vi "DataSelectNew.vi"(8 "error in (no error)":errorcluster, 9 "Table":string, 11 "Machine":string) -> (2 "error out":errorcluster)   [LabVIEW 2012]
uses:
  <vilib>/addons/database/Auxilliary.llb/DB Tools Cursor Type.ctl
  Global1.vi
  <vilib>/addons/database/Connection.llb/DB Tools Open Connec (Path).vi
  <vilib>/addons/database/Connection.llb/Conn Execute.vi
  <vilib>/addons/database/Recordset.llb/Rec Fetch Integer Data (R).vi
  <vilib>/addons/database/Recordset.llb/Rec Destroy - Connection.vi
  <vilib>/addons/database/_DB Variant To Data/Database Variant To Data.xnode
  <vilib>/addons/database/NI_Database_API.lvlib
panel:
  out "concatenated string 3":string
  out "error out 3":errorcluster
  out "data 3":i32
  out "concatenated string 2":string
  out "x > y?":bool
  out "concatenated string":string
  in  "input cluster":T1
  out "sum 2":i32
  in  "input cluster 2":T1
  out "sum":i32
  out "x = y? 2":bool
  out "element":i32
  out "data 2":string
  out "x = y?":bool
  out "data":variant[][](array[variant])
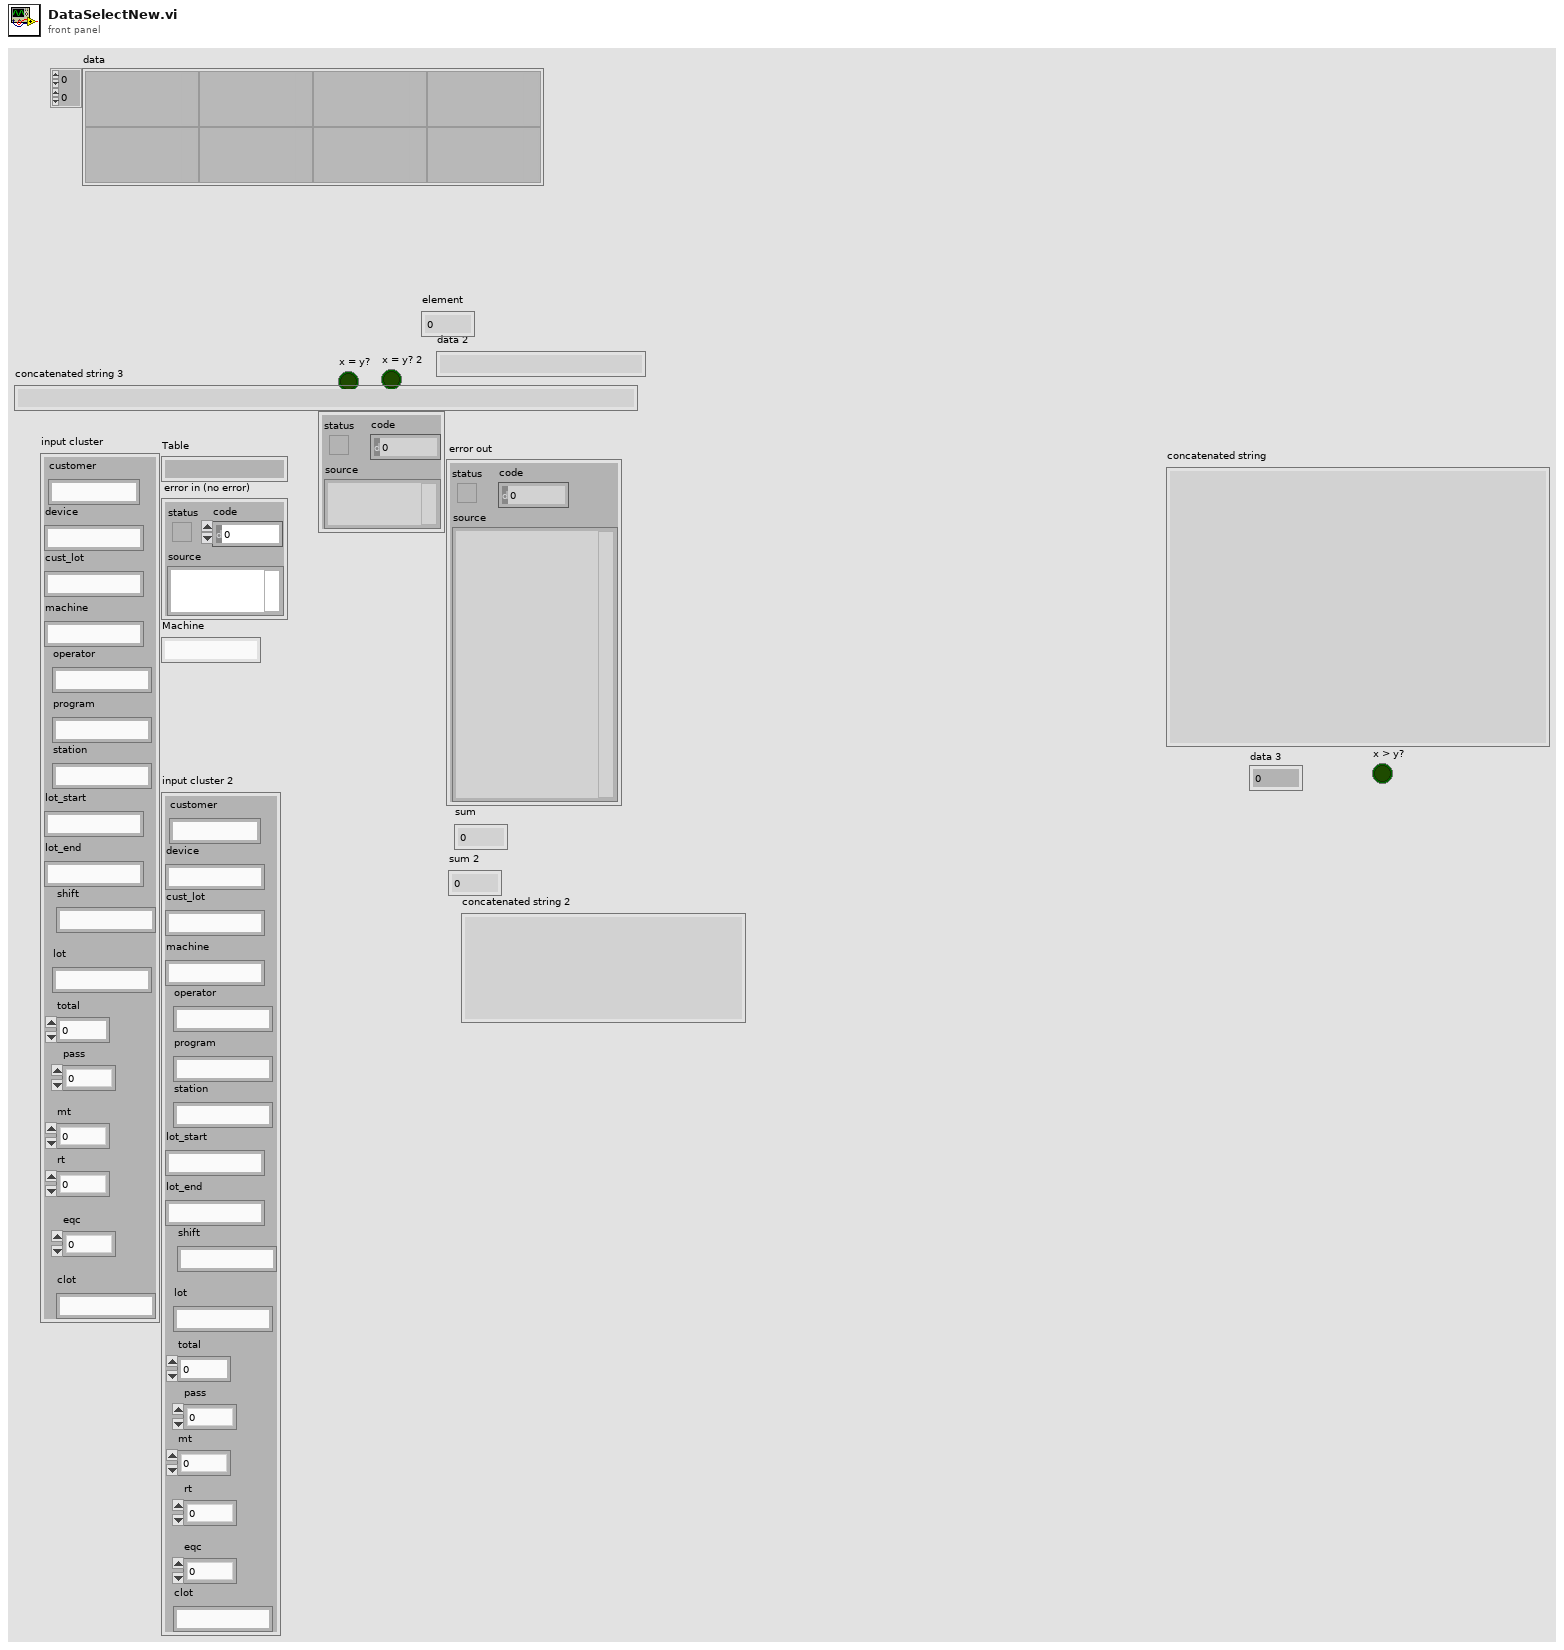
[diagram p1: front panel]
types:
  T1 = cluster{"customer":string, "device":string, "cust_lot":string, "machine":string, "operator":string, "program":string, "station":string, "lot_start":string, "lot_end":string, "shift":string, "lot":string, "total":dbl, "pass":dbl, "mt":dbl, "rt":dbl, "eqc":dbl, "clot":string}
  T2 = typedef "NI_Database_API.lvlib/Conn ObjectReference.ctl" = refnum<k1>
  T3 = typedef "NI_Database_API.lvlib/DB Tools Cursor Type.ctl" = enum16{"forward-only", "keyset", "dynamic", "static"}
  T4 = typedef "NI_Database_API.lvlib/Rec ObjectReference.ctl" = refnum<k1>
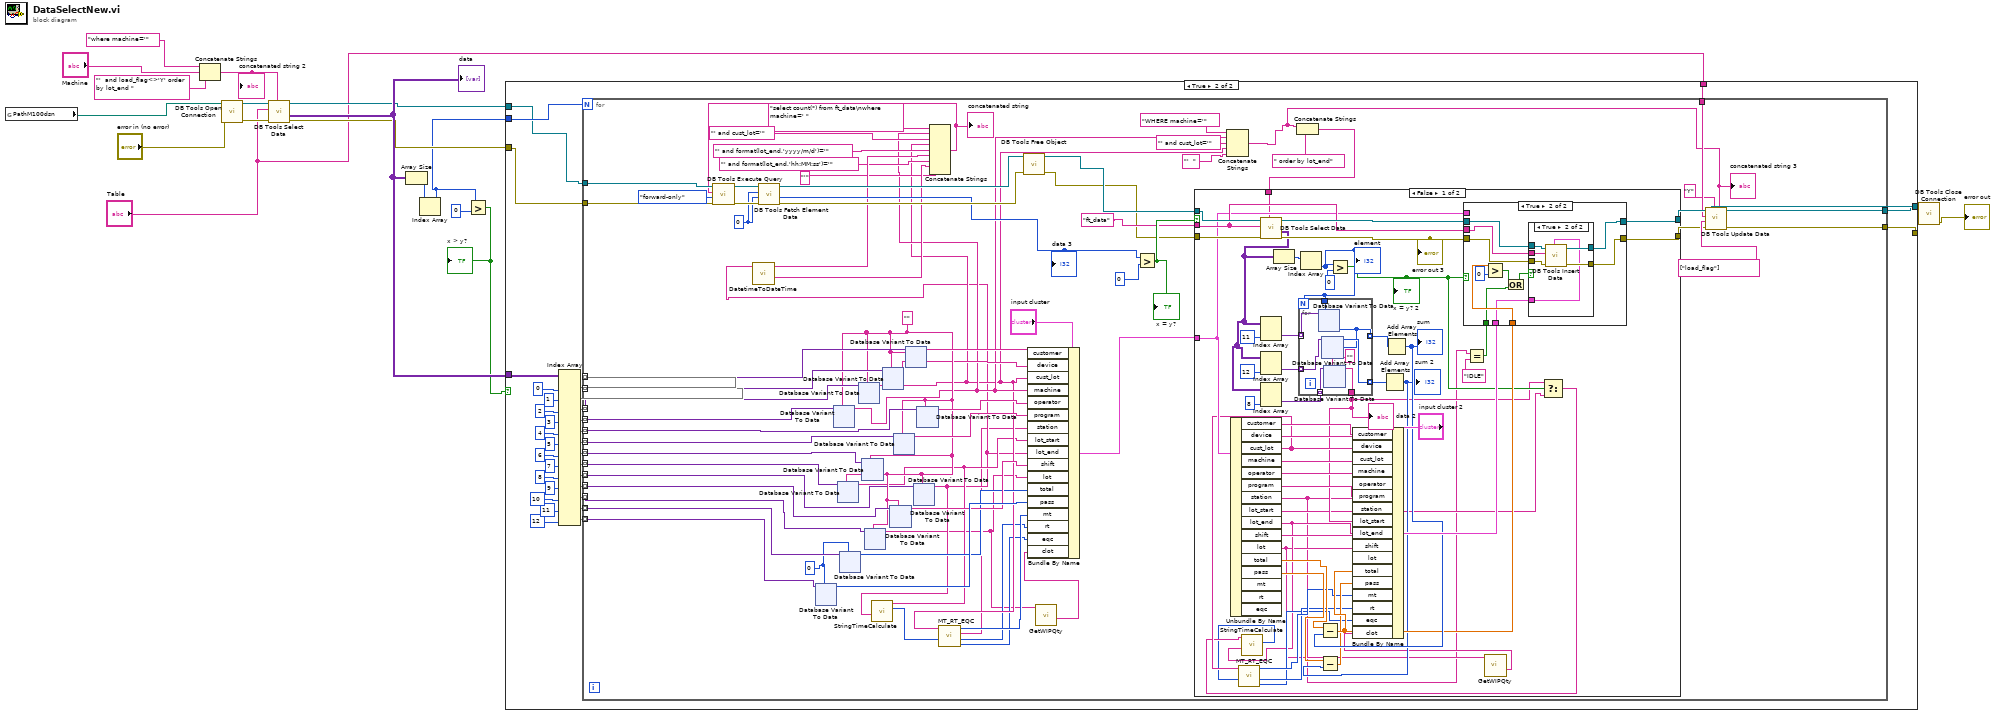
[diagram p0: block diagram]
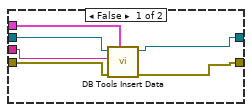
[diagram p3: hidden frame]
diagram:
  n1 = global read "Global1.vi" "PathM100dsn"() -> (w1:path)
  n2 = Concatenate Strings("where machine='" ("string"), "Machine", "'  and load_flag<>'Y' order by lot_end " ("string")) -> (w8:string)
  "concatenated string 2" <- w8
  n3 = call-poly <vilib>:"DB Tools Open Connection.vi"("error in (no error)"="error in (no error)", "connection information"=w1) -> ("error out"=w17:errorcluster, "connection reference"=w18:T2)  [unwired: 6 in]
  n4 = call <vilib>:"DB Tools Select Data.vi"("condition"=w8, "error in (no error)"=w17, "table"="Table", "connection reference"=w18) -> ("error out"=w5:errorcluster, "data"=w15:variant[][], "connection reference out"=w6:T2)  [unwired: 2 in]
  "data" <- w15
  n5 = Array Size(array=w15) -> (size(s)=w16:i32[])
  n6 = Index Array(array=w16) -> (element=w4:i32)  [unwired: 1 in]
  n7 = Greater?(x=w4, y=0) -> (0:w3:bool)
  "x > y?" <- w3
  n8 = case shown="True" w3 {
    tunnel: w15 -> [_ w52]
    tunnel: [w20 w22] -> w14
    tunnel: [w19 w21] -> _
    tunnel: w6 -> [w20 w25]
    tunnel: w5 -> [w19 w24]
    tunnel: w4 -> [_ w26]
    tunnel: "Table" -> [_ w23]
    frame False {
    }
    frame True {
      n9 = Index Array(array=w52, index (col) #1=0 ("disabled index (col)"), index (col) #2=1 ("index (col)"), index (col) #3=2 ("index (col)"), index (col) #4=3 ("index (col)"), index (col) #5=4 ("index (col)"), index (col) #6=5 ("index (col)"), index (col) #7=6 ("index (col)"), index (col) #8=7 ("index (col)"), index (col) #9=8 ("index (col)"), index (col) #10=9 ("index (col)"), index (col) #11=10 ("index (col)"), index (col) #12=11 ("index (col)"), index (col) #13=12 ("index (col)")) -> (element #1=w39:variant[], element #2=w38:variant[], element #3=w37:variant[], element #4=w36:variant[], element #5=w35:variant[], element #6=w34:variant[], element #7=w33:variant[], element #8=w32:variant[], element #9=w31:variant[], element #10=w30:variant[], element #11=w29:variant[], element #12=w28:variant[], element #13=w27:variant[])  [unwired: 13 in]
      n10 = for {
        N: w26 -> [_]
        tunnel: w25 -> [w97]
        tunnel: w39 -> [w122] mode=indexing
        tunnel: w38 -> [w121] mode=indexing
        tunnel: w37 -> [w120] mode=indexing
        tunnel: w36 -> [w119] mode=indexing
        tunnel: w35 -> [w110] mode=indexing
        tunnel: w34 -> [w118] mode=indexing
        tunnel: w33 -> [w117] mode=indexing
        tunnel: w32 -> [w116] mode=indexing
        tunnel: w31 -> [w81] mode=indexing
        tunnel: w30 -> [w115] mode=indexing
        tunnel: w29 -> [w114] mode=indexing
        tunnel: w28 -> [w113] mode=indexing
        tunnel: w27 -> [w112] mode=indexing
        tunnel: w24 -> [w89]
        tunnel: w23 -> [w70]
        tunnel: [w68] -> w22
        tunnel: [w67] -> w21
        w90 = 0
        w111 = 0
        w104 = ""
        n11 = xnode "Database Variant To Data"("database variant"=w112, "type"=w111) -> ("data"=w106:i32)  [unwired: 1 in, 1 out]
        n12 = xnode "Database Variant To Data"("database variant"=w119, "type"=w104) -> ("data"=w75:string)  [unwired: 1 in, 1 out]
        n13 = xnode "Database Variant To Data"("database variant"=w116, "type"=w104) -> ("data"=w62:string)  [unwired: 1 in, 1 out]
        n14 = xnode "Database Variant To Data"("database variant"=w113, "type"=w111) -> ("data"=w98:i32)  [unwired: 1 in, 1 out]
        n15 = xnode "Database Variant To Data"("database variant"=w120, "type"=w104) -> ("data"=w66:string)  [unwired: 1 in, 1 out]
        n16 = xnode "Database Variant To Data"("database variant"=w117, "type"=w104) -> ()  [unwired: 1 in, 2 out]
        n17 = xnode "Database Variant To Data"("database variant"=w114, "type"=w104) -> ("data"=w55:string)  [unwired: 1 in, 1 out]
        n18 = xnode "Database Variant To Data"("database variant"=w121, "type"=w104) -> ("data"=w100:string)  [unwired: 1 in, 1 out]
        n19 = xnode "Database Variant To Data"("database variant"=w115, "type"=w104) -> ("data"=w99:string)  [unwired: 1 in, 1 out]
        n20 = xnode "Database Variant To Data"("database variant"=w118, "type"=w104) -> ("data"=w107:string)  [unwired: 1 in, 1 out]
        n21 = xnode "Database Variant To Data"("database variant"=w122, "type"=w104) -> ("data"=w109:string)  [unwired: 1 in, 1 out]
        n22 = xnode "Database Variant To Data"("database variant"=w81, "type"=w104) -> ("data"=w61:string)  [unwired: 1 in, 1 out]
        n23 = call "DatetimeToDateTime.vi"("Datetime string"=w61) -> ("Time string"=w78:string, "Date string"=w80:string)  [unwired: 9 in]
        n24 = call "StringTimeCalculate.vi"("End Date"=w61, "Start Date"=w62) -> ("Minutes"=w60:i32)  [unwired: 9 in]
        n25 = xnode "Database Variant To Data"("database variant"=w110, "type"=w104) -> ("data"=w108:string)  [unwired: 1 in, 1 out]
        n26 = Concatenate Strings("select count(*) from ft_data\nwhere machine=' " ("SQL query"), w75, "' and cust_lot='" ("string"), w66, "' and format(lot_end,'yyyy/m/d')='" ("string"), w80, "' and format(lot_end,'hh:MM:ss')='" ("string"), w78, "'" ("string")) -> (w93:string)
        "concatenated string" <- w93
        n27 = call-poly <vilib>:"DB Tools Execute Query.vi"("error in (no error)"=w89, "cursor type"=DB_Tools_Cursor_Type."forward-only", "SQL query"=w93, "connection reference"=w97) -> ("error out"=w91:errorcluster, "recordset reference"=w92:T4)  [unwired: 4 in]
        n28 = call-poly <vilib>:"DB Tools Fetch Element Data.vi"("error in (no error)"=w91, "type"=w90, "column index"=w90, "recordset reference"=w92) -> ("error out"=w85:errorcluster, "data"=w84:i32, "recordset reference out"=w88:T4)  [unwired: 3 in]
        "data 3" <- w84
        n29 = call "MT_RT_EQC.vi"("Data"=w60, "input string"=w66) -> ("EQC"=w63:i32, "RT"=w64:i32, "Station"=w56:string, "MT"=w65:i32)  [unwired: 6 in]
        n30 = call-poly <vilib>:"DB Tools Free Object.vi"("error in (no error)"=w85, "recordset reference"=w88) -> ("error out"=w86:errorcluster, "connection reference"=w87:T2)  [unwired: 8 in]
        n31 = call "GetWIPQty.vi"("Lotno"=w55) -> ("lotno"=w54:string)  [unwired: 6 in, 4 out]
        n32 = Bundle By Name(cluster="input cluster", "customer"=w109, "device"=w100, "cust_lot"=w66, "machine"=w75, "operator"=w108, "program"=w107, "station"=w56, "lot_start"=w62, "lot_end"=w61, "shift"=w99, "lot"=w55, "total"=w98, "pass"=w106, "mt"=w65, "rt"=w64, "eqc"=w63, "clot"=w54) -> (w101:T1)
        n33 = Greater?(x=w84, y=0) -> (0:w103:bool)
        "x = y?" <- w103
        n34 = Concatenate Strings("WHERE machine='" ("string"), w75, "' and cust_lot='" ("string"), w66, "'  " ("string")) -> (w57:string)
        "concatenated string 3" <- w57
        n35 = Concatenate Strings(w57, " order by lot_end" ("string")) -> (w58:string)
        n36 = case shown="False" w103 {
          tunnel: w87 -> [w173 w304]
          tunnel: w86 -> [w172 w303]
          tunnel: "ft_data" ("table") -> [w151 _]
          tunnel: w101 -> [w150 _]
          tunnel: [w164 w304] -> w71
          tunnel: [w163 w303] -> w72
          tunnel: w58 -> [w139 _]
          frame False {
            n37 = Unbundle By Name(w150) -> ("customer"=w141:string, "device"=w158:string, "cust_lot"=w138:string, "machine"=w157:string, "operator"=w156:string, "program"=w155:string, "station"=w126:string, "lot_start"=w131:string, "lot_end"=w134:string, "shift"=w154:string, "lot"=w128:string, "total"=w149:dbl, "pass"=w146:dbl)  [unwired: 3 out]
            n38 = call <vilib>:"DB Tools Select Data.vi"("condition"=w139, "error in (no error)"=w172, "table"=w151, "connection reference"=w173) -> ("error out"=w169:errorcluster, "data"=w143:variant[][], "connection reference out"=w170:T2)  [unwired: 2 in]
            "error out 3" <- w169
            n39 = Index Array(array=w143, index (col)=11) -> (element=w166:variant[])  [unwired: 1 in]
            n40 = Index Array(array=w143, index (col)=12) -> (element=w160:variant[])  [unwired: 1 in]
            n41 = Index Array(array=w143, index (col)=8 ("disabled index (col)")) -> (element=w140:variant[])  [unwired: 1 in]
            n42 = Array Size(array=w143) -> (size(s)=w171:i32[])
            n43 = Index Array(array=w171) -> (element=w165:i32)  [unwired: 1 in]
            "element" <- w165
            n44 = for {
              N: w165 -> [_]
              tunnel: w166 -> [w181] mode=indexing
              tunnel: w165 -> [w180]
              tunnel: [w177] -> w162 mode=indexing
              tunnel: w160 -> [w179] mode=indexing
              tunnel: [w178] -> w159 mode=indexing
              tunnel: w140 -> [w176] mode=indexing
              tunnel: [w174] -> w132
              n45 = xnode "Database Variant To Data"("database variant"=w181, "type"=w180) -> ("data"=w177:i32)  [unwired: 1 in, 1 out]
              n46 = xnode "Database Variant To Data"("database variant"=w179, "type"=w177) -> ("data"=w178:i32)  [unwired: 1 in, 1 out]
              n47 = xnode "Database Variant To Data"("database variant"=w176, "type"="") -> ("data"=w174:string)  [unwired: 1 in, 1 out]
            }
            "data 2" <- w132
            n48 = Greater?(x=w165, y=0) -> (0:w133:bool)
            "x = y? 2" <- w133
            n49 = Add Array Elements(numeric array=w159) -> (sum=w145:i32)
            "sum 2" <- w145
            n50 = Subtract(x=w146, y=w145) -> (x-y=w144:dbl)
            n51 = Add Array Elements(numeric array=w162) -> (sum=w148:i32)
            "sum" <- w148
            n52 = Subtract(x=w149, y=w148) -> (x-y=w147:dbl)
            n53 = Equal?(x=w126, y="IDLE") -> (x = y?=w124:bool)
            n54 = call "GetWIPQty.vi"("Lotno"=w128) -> ("lotno"=w127:string)  [unwired: 6 in, 4 out]
            n55 = Select(t=w132, s=w133, f=w131) -> (s? t:f=w130:string)
            n56 = call "StringTimeCalculate.vi"("End Date"=w134, "Start Date"=w130) -> ("Minutes"=w129:i32)  [unwired: 9 in]
            n57 = call "MT_RT_EQC.vi"("Data"=w129, "input string"=w138) -> ("EQC"=w135:i32, "RT"=w136:i32, "MT"=w137:i32)  [unwired: 6 in, 1 out]
            n58 = Bundle By Name(cluster="input cluster 2", "customer"=w141, "device"=w158, "cust_lot"=w138, "machine"=w157, "operator"=w156, "program"=w155, "station"=w126, "lot_start"=w132, "lot_end"=w134, "shift"=w154, "lot"=w128, "total"=w147, "pass"=w144, "mt"=w137, "rt"=w136, "eqc"=w135, "clot"=w127) -> (w152:T1)
            n59 = case shown="True" w133 {
              tunnel: w170 -> [w283 w292]
              tunnel: w169 -> [w282 w291]
              tunnel: [w281 w289] -> w164
              tunnel: [w280 w288] -> w163
              tunnel: w152 -> [_ w287]
              tunnel: w151 -> [w279 w290]
              tunnel: w150 -> [w278 _]
              tunnel: w147 -> [_ w293]
              tunnel: w124 -> [_ w284]
              frame False {
                n60 = call <vilib>:"DB Tools Insert Data.vi"("data"=w278, "error in (no error)"=w282, "table"=w279, "connection reference"=w283) -> ("error out"=w280:errorcluster, "connection reference out"=w281:T2)  [unwired: 6 in]
              }
              frame True {
                n61 = Greater?(x=w293, y=0) -> (0:w285:bool)
                n62 = Or(x=w285, y=w284) -> (x .or. y?=w286:bool)
                n63 = case shown="True" w286 {
                  tunnel: w292 -> [w296 w302]
                  tunnel: w291 -> [w295 w301]
                  tunnel: w290 -> [_ w300]
                  tunnel: [w296 w299] -> w289
                  tunnel: [w295 w298] -> w288
                  tunnel: w287 -> [_ w297]
                  frame False {
                  }
                  frame True {
                    n64 = call <vilib>:"DB Tools Insert Data.vi"("data"=w297, "error in (no error)"=w301, "table"=w300, "connection reference"=w302) -> ("error out"=w298:errorcluster, "connection reference out"=w299:T2)  [unwired: 6 in]
                  }
                }
              }
            }
          }
          frame True {
          }
        }
        n65 = call <vilib>:"DB Tools Update Data.vi"("condition"=w57, "data"="Y", "error in (no error)"=w72, "columns"=string[] ["load_flag"], "table"=w70, "connection reference"=w71) -> ("error out"=w67:errorcluster, "connection reference out"=w68:T2)  [unwired: 4 in]
      }
    }
  }
  n66 = call <vilib>:"DB Tools Close Connection.vi"("connection reference"=w14) -> ("error out"=→"error out":errorcluster)  [unwired: 6 in]
